vi "Shooter Controller.vi"(8 "error in":errorcluster) -> ()   [LabVIEW 2019]
doc: "This VI executes continuously carrying out the current operation and responding to updates or new operations. It will often contain the timing or control code that is difficult to place directly in TeleOp. This VI generally opens all sensors and motors and isolates the rest of the robot code from knowing how the operations are carried out."
uses:
  <vilib>/Rock Robotics/WPI/Framework/Completion Status.ctl
  Shooter Setpoints.ctl
  Shooter Operations.ctl
  <vilib>/Rock Robotics/WPI/ThirdParty/REV Robotics/SPARK MAX/Typedef/Spark MAX Idle Mode.ctl
  <vilib>/Rock Robotics/WPI/ThirdParty/REV Robotics/SPARK MAX/Typedef/Spark MAX Control Type.ctl
  <vilib>/Rock Robotics/Network Tables/NT Write Number.vi
  <vilib>/Rock Robotics/Network Tables/NT Write Boolean.vi
panel:
  out "?":dbl
  out "flywheel":dbl
  out "tx":dbl
  in  "Interactive Values":T1
  out "Current\nCmd":string
  in  "Buttons":cluster{"Execute Cmd":bool, "Abort Cmd":bool}
  out "Command Timing":cluster{"Start Time (ms)":u32, "Iterations":i32}
  out "Status":T3
  # "Tip: It may be helpful to observe inputs and sensor values.\nYou may also want to display tuning or debugging controls."
  # "Interactive Command: You may fill in the settings for a command\nand schedule it with the Execute button. You can observe and abort\nany command while fine tuning the code for the controller."
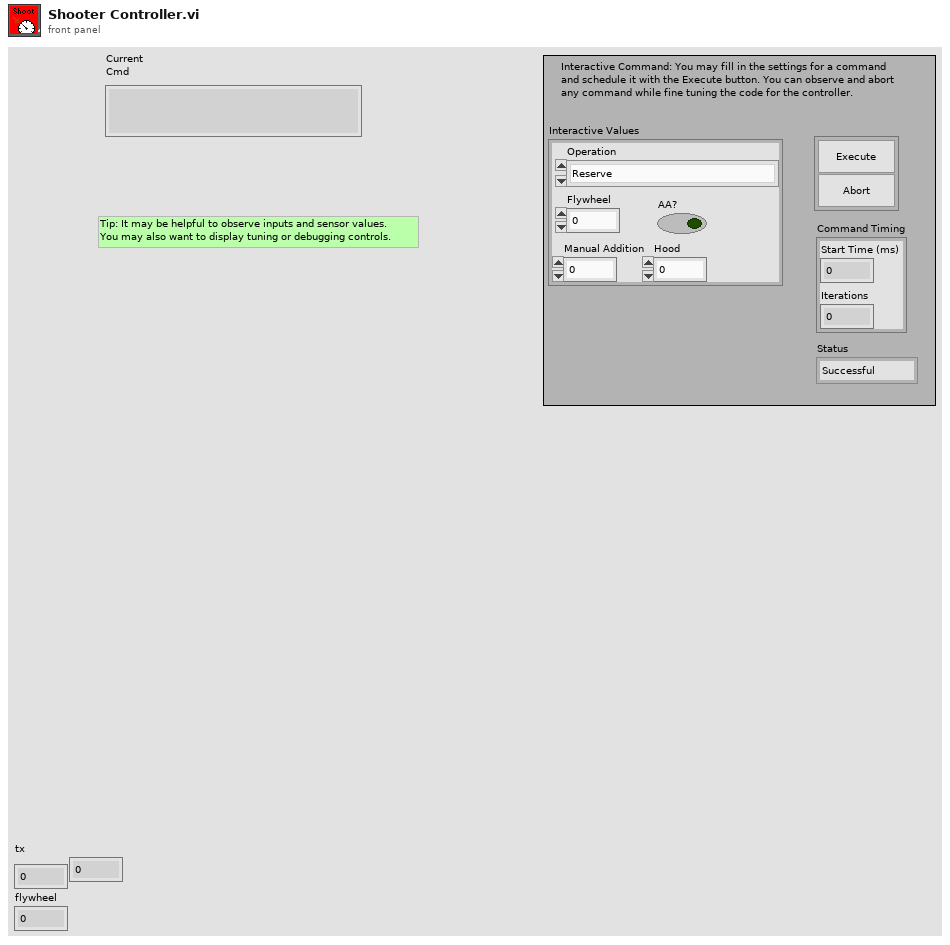
[diagram p1: front panel]
types:
  T1 = typedef "Shooter Setpoints.ctl" = cluster{"Operation":T2, "Flywheel":dbl, "Hood":dbl, "AA?":bool, "Manual Addition":dbl}
  T2 = typedef "Shooter Operations.ctl" = enum16{"Reserve", "Read Current", "Immediate", "Shoot"}
  T3 = typedef "Completion Status.ctl" = enum16{"Successful", "Aborted", "Incomplete"}
  T4 = typedef "Spark MAX Idle Mode.ctl" = enum16{"Coast", "Brake"}
  T5 = typedef "WPI_MotorControlDeviceRef.ctl" = cluster{"DeviceStatus":errorcluster, "Type":T6, "PWM":cluster{"PWM Channel":T7, "DeadBand":T8}, "CAN":cluster{"Device Number":u8, "SetOutput VI Ref":variant, "GetOutput VI Ref":variant, "Enable VI Ref":variant, "Disable VI Ref":variant, "Data":variant}, "Invert":bool, "DIO PWM":cluster{"PWM \"Enable\" Channel":T7, "DIOChannel":T9, "PWM Rate":dbl}}
  T6 = typedef "WPI_MotorControlType.ctl" = enum16{"PWM", "CAN", "DIO PWM"}
  T7 = typedef "FPGA_DIOPWMChannel.ctl" = enum8{"PWM 0", "PWM 1", "PWM 2", "PWM 3", "PWM 4", "PWM 5", "PWM 6", "PWM 7", "PWM 8", "PWM 9", "PWM MXP 0", "PWM MXP 1", "PWM MXP 2", "PWM MXP 3", "PWM MXP 4", "PWM MXP 5", "PWM MXP 6", "PWM MXP 7", "PWM MXP 8", "PWM MXP 9", "Invalid"}
  T8 = typedef "WPI_PWMDeadband.ctl" = cluster{"Name":string, "maxPositivePwm":i32, "minPositivePwm":i32, "centerPwm":i32, "maxNegativePwm":i32, "minNegativePwm":i32, "angularRange":u16}
  T9 = typedef "FPGA_DIOChannel.ctl" = enum8{"DIO 0", "DIO 1", "DIO 2", "DIO 3", "DIO 4", "DIO 5", "DIO 6", "DIO 7", "DIO 8", "DIO 9", "DIO MXP 0", "DIO MXP 1", "DIO MXP 2", "DIO MXP 3", "DIO MXP 4", "DIO MXP 5", "DIO MXP 6", "DIO MXP 7", "DIO MXP 8", "DIO MXP 9", "DIO MXP 10", "DIO MXP 11", "DIO MXP 12", "DIO MXP 13", "DIO MXP 14", "DIO MXP 15", "SPI Port CS1", "SPI Port CS2", "SPI Port CS3", "SPI Port MISO", "SPI Port MOSI", "Invalid"}
  T10 = typedef "Command Status Info.ctl" = cluster{"Name":string, "Status":T3, "notifier out":T11}
  T11 = typedef "Completion Notifier.ctl" = refnum<notifier>
  T12 = cluster{"Current Command":T1, "Command Timing":cluster{"Start Time (ms)":u32, "Iterations":i32}, "Command Arguments":cluster{"Command Info":T10, "Description":string, "Default Command":T1, "queue out":refnum<queue>, "Subsystem Name":string}}
  T13 = cluster{"P Gain":dbl, "I Gain":dbl, "D Gain":dbl, "F Gain":dbl, "I Zone":dbl, "Min Output":dbl, "Max Output":dbl}
  T14 = typedef "Spark MAX Control Type.ctl" = enum16{"Percent VBus", "Voltage", "Velocity", "Position", "Smart Motion", "Current", "Smart Velocity"}
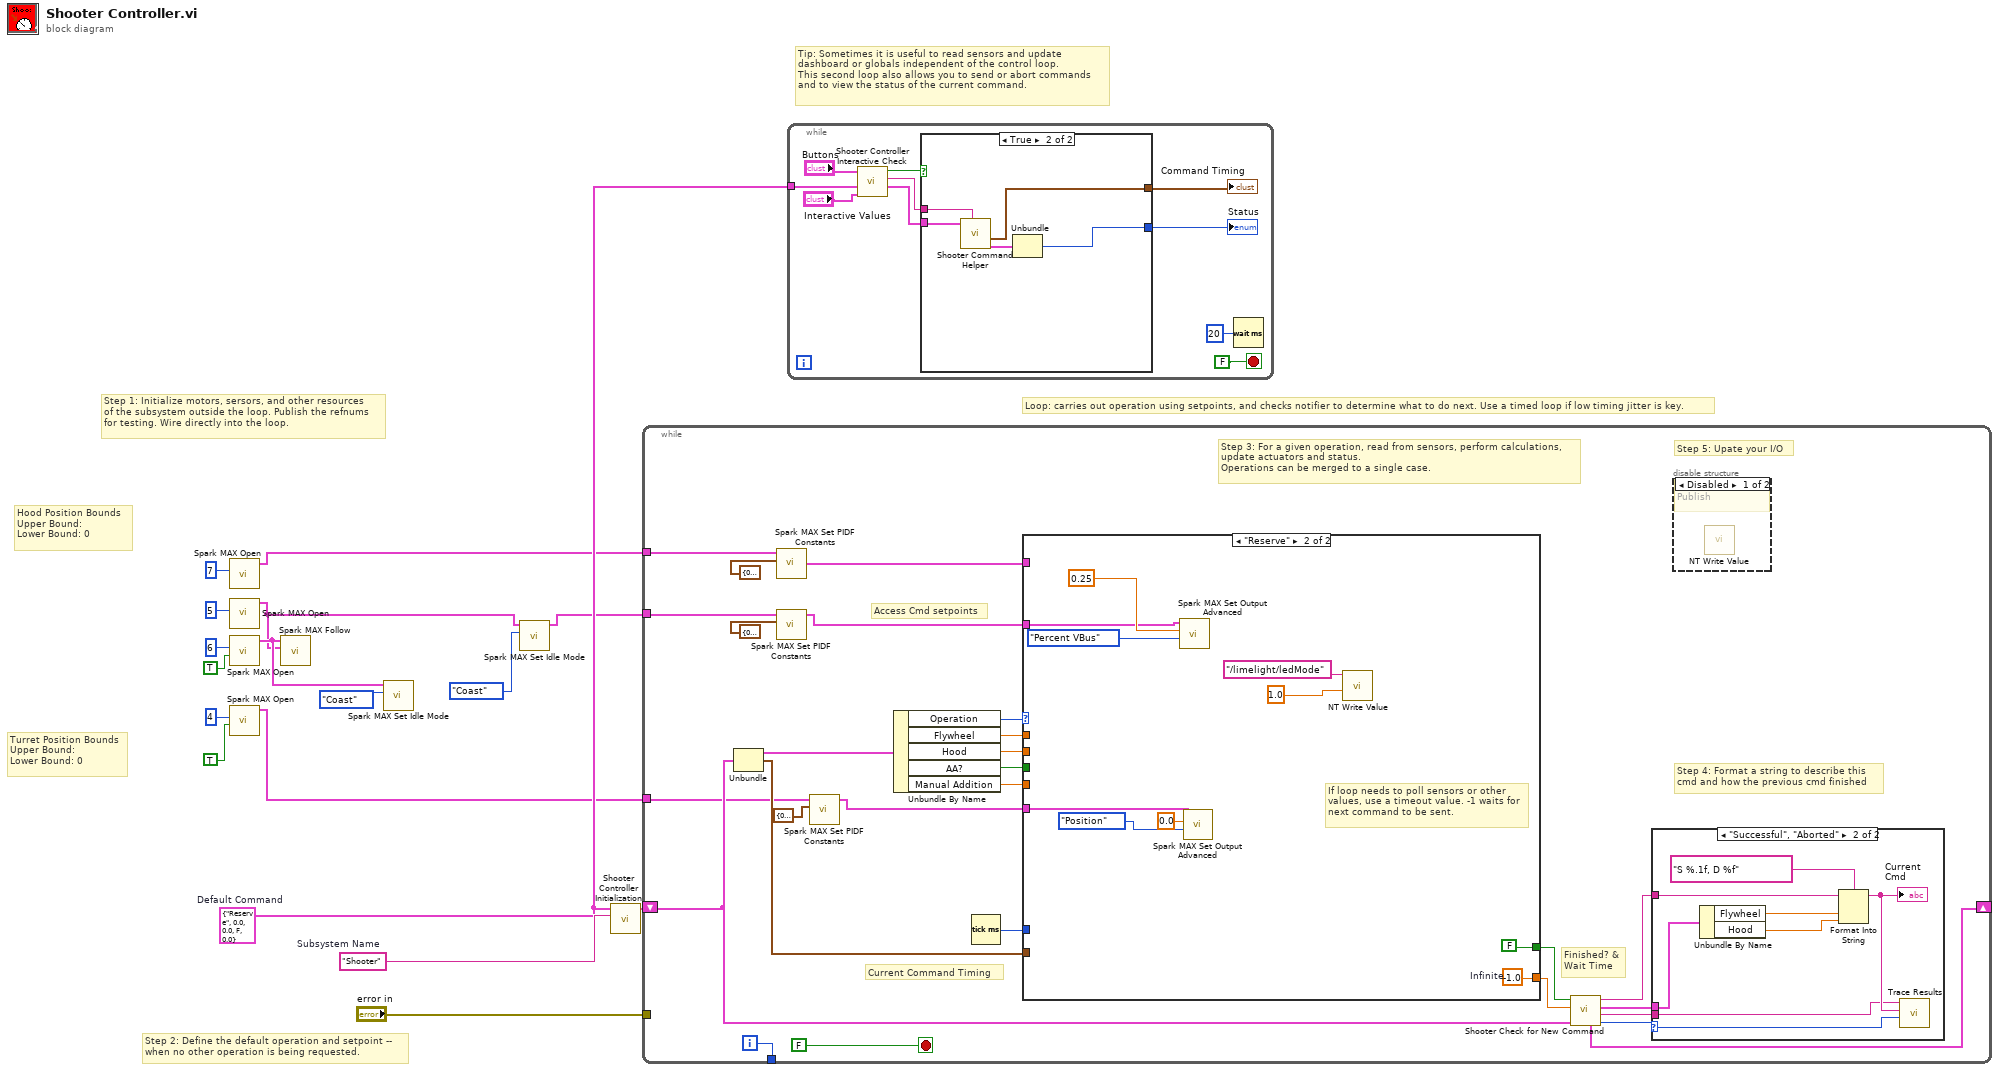
[diagram p0: block diagram]
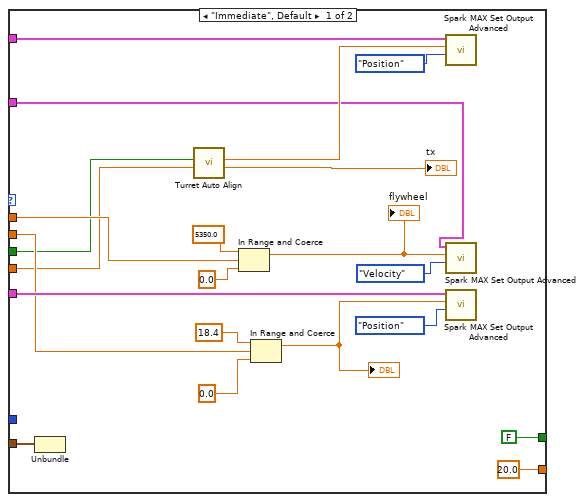
[diagram p2: hidden frame]
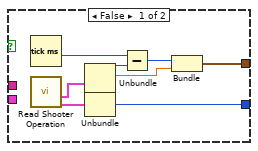
[diagram p5: hidden frame]
diagram:
  w14 = T1 {"Operation"=enum."Reserve", "Flywheel"=0.0, "Hood"=0.0, "AA?"=FALSE, "Manual Addition"=0.0}  # Default Command
  w15 = "Shooter"  # Subsystem Name
  # "Turret Position Bounds\nUpper Bound:\nLower Bound: 0"
  # "Hood Position Bounds\nUpper Bound:\nLower Bound: 0"
  # "Tip: Sometimes it is useful to read sensors and update\ndashboard or globals independent of the control loop.\nThis second loop also allows you to send or abort commands\nand to view the status of the current command."
  # "Step 2: Define the default operation and setpoint --\nwhen no other operation is being requested."
  # "Step 1: Initialize motors, sersors, and other resources\nof the subsystem outside the loop. Publish the refnums\nfor testing. Wire directly into the loop."
  # "Loop: carries out operation using setpoints, and checks notifier to determine what to do next. Use a timed loop if low timing jitter is key."
  n1 = call <vilib>:"Spark MAX Open.vi"("Device Number"=u8 7) -> ("MotorControlDeviceRef"=w4:T5)  [unwired: 9 in, 1 out]
  n2 = call <vilib>:"Spark MAX Open.vi"("Device Number"=u8 5) -> ("MotorControlDeviceRef"=w2:T5)  [unwired: 9 in, 1 out]
  n3 = call <vilib>:"Spark MAX Open.vi"("Invert"=TRUE, "Device Number"=u8 6) -> ("MotorControlDeviceRef"=w6:T5)  [unwired: 8 in, 1 out]
  n4 = call <vilib>:"Spark MAX Open.vi"("Invert"=TRUE, "Device Number"=u8 4) -> ("MotorControlDeviceRef"=w3:T5)  [unwired: 8 in, 1 out]
  n5 = call <vilib>:"Spark MAX Follow.vi"("Master Controller"=w2, "MotorControlDeviceRef"=w6) -> ()  [unwired: 8 in, 2 out]
  n6 = call <vilib>:"Spark MAX Set Idle Mode.vi"("Idle Mode"=Spark_MAX_Idle_Mode."Coast", "MotorControlDeviceRef in"=w6) -> ()  [unwired: 8 in, 2 out]
  n7 = call <vilib>:"Spark MAX Set Idle Mode.vi"("Idle Mode"=Spark_MAX_Idle_Mode."Coast", "MotorControlDeviceRef in"=w2) -> ("MotorControlDeviceRef out"=w1:T5)  [unwired: 8 in, 1 out]
  n8 = call "Shooter Controller Initialization.vi"("Subsystem Name"=w15, "Default Command"=w14) -> ("Current Command"=w16:T12)  [unwired: 9 in]
  n9 = while {
    shift-right: [w37] -> _
    shift-left: w16 -> [w30]
    tunnel: [w43] -> _
    tunnel: "error in" -> [_]
    tunnel: w1 -> [w25]
    tunnel: w4 -> [w23]
    tunnel: w3 -> [w19]
    i -> [w43]
    stop <- FALSE stop-if-true
    # "Step 5: Upate your I/O"
    # "Step 4: Format a string to describe this\ncmd and how the previous cmd finished"
    # "Current Command Timing"
    # "Access Cmd setpoints"
    # "Finished? &\nWait Time"
    # "Step 3: For a given operation, read from sensors, perform calculations,\nupdate actuators and status.\nOperations can be merged to a single case."
    n10 = Unbundle(w30) -> ("Current Command"=w42:T1, "Command Timing"=w39:cluster{"Start Time (ms)":u32, "Iterations":i32})  [unwired: 1 out]
    n11 = call <vilib>:"Spark MAX Set PIDF Constants.vi"("PID Constants"=T13 {"P Gain"=0.06, "I Gain"=0.0, "D Gain"=0.0, "F Gain"=0.0, "I Zone"=0.0, "Min Output"=-1.0, "Max Output"=1.0} ("Turret PID"), "MotorControlDeviceRef"=w23) -> ("MotorControlDeviceRef"=w22:T5)  [unwired: 8 in, 1 out]
    n12 = call <vilib>:"Spark MAX Set PIDF Constants.vi"("PID Constants"=T13 {"P Gain"=0.0002, "I Gain"=0.0, "D Gain"=0.0, "F Gain"=0.00018, "I Zone"=0.0, "Min Output"=-1.0, "Max Output"=1.0} ("Flywheel PID"), "MotorControlDeviceRef"=w25) -> ("MotorControlDeviceRef"=w21:T5)  [unwired: 8 in, 1 out]
    n13 = call <vilib>:"Spark MAX Set PIDF Constants.vi"("PID Constants"=T13 {"P Gain"=0.13, "I Gain"=0.0, "D Gain"=0.0, "F Gain"=0.0, "I Zone"=0.0, "Min Output"=-1.0, "Max Output"=1.0} ("Hood PID"), "MotorControlDeviceRef"=w19) -> ("MotorControlDeviceRef"=w18:T5)  [unwired: 8 in, 1 out]
    n14 = Unbundle By Name(w42) -> ("Operation"=w41:T2, "Flywheel"=w38:dbl, "Hood"=w29:dbl, "AA?"=w28:bool, "Manual Addition"=w27:dbl)
    n15 = Tick Count (ms)() -> (millisecond timer value=w40:u32)
    n16 = case shown="\"Reserve\"" w41 {
      tunnel: [20.0 ("Wait ms") w75] -> w35
      tunnel: [FALSE ("ignore previous (F)") FALSE ("ignore previous (F)")] -> w36
      tunnel: w39 -> [w64 _]
      tunnel: w40 -> [_ _]
      tunnel: w38 -> [w52 _]
      tunnel: w22 -> [w50 _]
      tunnel: w18 -> [w53 w73]
      tunnel: w29 -> [w51 _]
      tunnel: w28 -> [w49 _]
      tunnel: w27 -> [w47 _]
      tunnel: w21 -> [w45 w66]
      frame "Immediate", Default {
        n17 = Unbundle(w64) -> ()  [unwired: 2 out]
        n18 = call "Turret Auto Align.vi"("Manual Addition"=w47, "AA?"=w49) -> ("tx"=→"tx":dbl, "Turret New Position"=w48:dbl)  [unwired: 7 in, 1 out]
        n19 = In Range and Coerce(upper limit=5350.0, x=w52, lower limit=0.0) -> (coerced(x)=w58:dbl)  [unwired: 1 out]
        "flywheel" <- w58
        n20 = In Range and Coerce(upper limit=18.4, x=w51, lower limit=0.0) -> (coerced(x)=w59:dbl)  [unwired: 1 out]
        "?" <- w59
        n21 = call <vilib>:"Spark MAX Set Output Advanced.vi"("Control Mode"=Spark_MAX_Control_Type."Position", "Setpoint"=w48, "MotorControlDevRef"=w50) -> ()  [unwired: 7 in, 2 out]
        n22 = call <vilib>:"Spark MAX Set Output Advanced.vi"("Control Mode"=Spark_MAX_Control_Type."Velocity", "Setpoint"=w58, "MotorControlDevRef"=w45) -> ()  [unwired: 7 in, 2 out]
        n23 = call <vilib>:"Spark MAX Set Output Advanced.vi"("Control Mode"=Spark_MAX_Control_Type."Position", "Setpoint"=w59, "MotorControlDevRef"=w53) -> ()  [unwired: 7 in, 2 out]
      }
      frame "Reserve" {
        w75 = -1.0  # Infinite
        # "If loop needs to poll sensors or other\nvalues, use a timeout value. -1 waits for\nnext command to be sent."
        n24 = call <vilib>:"Spark MAX Set Output Advanced.vi"("Control Mode"=Spark_MAX_Control_Type."Percent VBus", "Setpoint"=0.25, "MotorControlDevRef"=w66) -> ()  [unwired: 7 in, 2 out]
        n25 = call <vilib>:"Spark MAX Set Output Advanced.vi"("Control Mode"=Spark_MAX_Control_Type."Position", "Setpoint"=0.0, "MotorControlDevRef"=w73) -> ()  [unwired: 7 in, 2 out]
        n26 = call-poly <vilib>:"NT Write Value.vi"("Numeric"=1.0, "Name"="/limelight/ledMode") -> ()  [unwired: 9 in, 1 out]
      }
    }
    n27 = call "Shooter Check for New Command.vi"("Current Command"=w30, "Wait time (ms)"=w35, "Finished?"=w36) -> ("Completion"=w31:T3, "Subsystem Name"=w32:string, "Current Command"=w33:T1, "Initial Trace String"=w34:string, "NextCommand"=w37:T12)  [unwired: 4 in]
    n28 = case shown="\"Successful\", \"Aborted\"" w31 {
      selector: w31 -> [_ w83]
      tunnel: w34 -> [_ w79]
      tunnel: w33 -> [_ w80]
      tunnel: w32 -> [_ w76]
      frame "Incomplete", Default {
        # "Continuing current command"
      }
      frame "Successful", "Aborted" {
        # "Report and setup for next command"
        n29 = Unbundle By Name(w80) -> ("Flywheel"=w82:dbl, "Hood"=w77:dbl)
        n30 = Format Into String(format string="S %.1f, D %f", initial string=w79, w82, w77) -> (resulting string=w78:string)  [unwired: 1 in, 1 out]
        "Current\nCmd" <- w78
        n31 = call <vilib>:"Trace Results.vi"("Status of previous command"=w83, "Description"=w78, "Subsystem"=w76) -> ()  [unwired: 9 in]
      }
    }
    n32 = disable-structure shown="Disabled" {
      frame Disabled {
        # "Publish"
        n33 = call-poly <vilib>:"NT Write Value.vi"() -> ()  [unwired: 11 in, 1 out]
      }
      frame Enabled {
      }
    }
  }
  n34 = while {
    tunnel: w14 -> [w90]
    stop <- FALSE stop-if-true
    n35 = call "Shooter Controller Interactive Check.vi"("Interactive Command in"="Interactive Values", "Default Command"=w90, "Buttons"="Buttons") -> ("Interactive Command out"=w87:T1, "Trace String"=w88:string, "Schedule"=w89:bool)  [unwired: 6 in]
    n36 = case shown="True" w89 {
      tunnel: [w101 w106] -> w86
      tunnel: w87 -> [_ w104]
      tunnel: [w97 w102] -> w85
      tunnel: w88 -> [_ w105]
      frame False {
        n37 = Tick Count (ms)() -> (millisecond timer value=w96:u32)
        n38 = call "Read Shooter Operation.vi"() -> ("Command Info"=w94:T10, "SubSystem Data"=w95:T1)  [unwired: 9 in, 1 out]
        n39 = Unbundle(w95) -> ("Operation"=w100:T2, "Flywheel"=w98:dbl)  [unwired: 3 out]
        n40 = Unbundle(w94) -> ("Status"=w101:T3)  [unwired: 2 out]
        n41 = Subtract(x=w96, y=w100) -> (x-y=w99:u32)
        n42 = Bundle(w99, "Flywheel"=w98) -> (w97:cluster{u32, "Flywheel":dbl})  [unwired: 1 in]
      }
      frame True {
        n43 = call "Shooter Command Helper.vi"("Description"=w105, "SubSystem Data"=w104) -> ("Command Info Out"=w103:T10, "Command Timing"=w102:cluster{"Start Time (ms)":u32, "Iterations":i32})  [unwired: 7 in, 1 out]
        n44 = Unbundle(w103) -> ("Status"=w106:T3)  [unwired: 2 out]
      }
    }
    "Status" <- w86
    "Command Timing" <- w85
    n45 = Wait (ms)(milliseconds to wait=u32 20) -> ()  [unwired: 1 out]
  }
